vi "Configure Car Wash Model.vi"(4 "iFan Controller Type":refnum<class "iFan Controller.lvclass">, 6 "Splash Screen Contract Model Type":refnum<class "iSplash Screen Contract Model.lvclass">, 8 "Process Builder Type":refnum<class "Test Executive Builder Model.lvclass">, 9 "Process Model Type":refnum<class "iProcess Model.lvclass">, 10 "Car Position Monitor Type":refnum<class "iCar Position Monitor Model.lvclass">, 11 "Car Wash Model in":refnum<class "Car Wash Model.lvclass">) -> (3 "Car Wash Model out":refnum<class "Car Wash Model.lvclass">)   [LabVIEW 2019, in "Car Wash Model.lvclass"]
uses:
  <vilib>/gpm_packages/@cs/Car-wash/Source/Car Wash Model/Car Wash Model/Car Wash Model.lvclass
  <vilib>/gpm_packages/@cs/Car-wash/Source/iCar Position Monitor Model/iCar Position Monitor Model/iCar Position Monitor Model.lvclass
  <vilib>/gpm_packages/@cs/Car-wash/Source/iProcess Model/iProcess Model/iProcess Model.lvclass
  <vilib>/gpm_packages/@cs/Car-wash/Source/iSplash Screen Contract Model/iSplash Screen Contract Model.lvclass
  <vilib>/gpm_packages/@cs/Test-executive-builder/Source/Test Executive Builder Model/Test Executive Builder Model/Test Executive Builder Model.lvclass
  <vilib>/gpm_packages/@cs/Car-wash/Source/iFan Controller/iFan Controller.lvclass
  <vilib>/gpm_packages/@cs/Car-wash/Source/Car Wash Model/Car Wash Model/Car Wash Model.lvclass/Car Wash Model.ctl
  <vilib>/gpm_packages/@cs/Car-wash/Source/Fan Controller Ref/Fan Controller Ref.lvclass
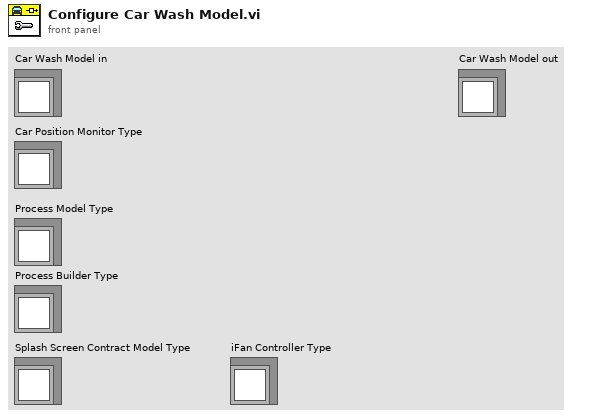
[diagram p1: front panel]
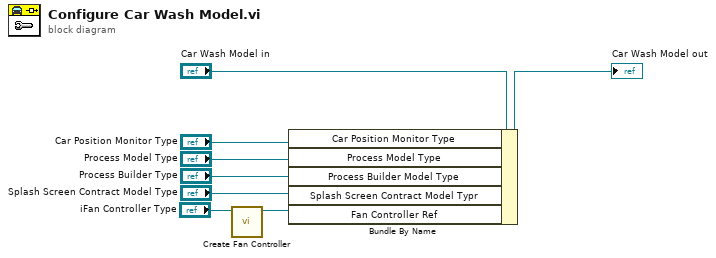
[diagram p0: block diagram]
diagram:
  n1 = call <vilib>:"Create Fan Controller.vi"("Fan Controller Type"="iFan Controller Type") -> ("Fan Controller Ref"=w1:refnum<data-value>)  [unwired: 9 in, 1 out]
  n2 = Bundle By Name(cluster="Car Wash Model in", "Car Position Monitor Type"="Car Position Monitor Type", "Process Model Type"="Process Model Type", "Process Builder Model Type"="Process Builder Type", "Splash Screen Contract Model Typr"="Splash Screen Contract Model Type", "Fan Controller Ref"=w1) -> (→"Car Wash Model out":refnum<class "Car Wash Model.lvclass">)
